vi "find_PrepLineObject_by_Name.vi"(9 "Name of Object":string, 10 "PrepLineObjects in":refnum<class "PrepLineObject.lvclass">[](array[class])) -> (0 "found PrepLineObject":refnum<class "PrepLineObject.lvclass">, 1 "instrument":string, 2 "selected array":bool[](array[boolean]), 3 "PrepLineObjectsOut":refnum<class "PrepLineObject.lvclass">[](array[class]), 4 "index of found":i32, 5 "found?":bool)   [LabVIEW 2017]
doc: "According to Name the correct PrepLineObject is located by looking through the Array of all PrepLineObjects (stored in a queue). The output array has the same size as the array with the switch objects and shows (state = true) the location of the Object that that has been selected. It also outputs the name of the instrument that belongs to the PrepLineObject that has changed"
uses:
  Classes/PrepLineObject/PrepLineObject.lvclass
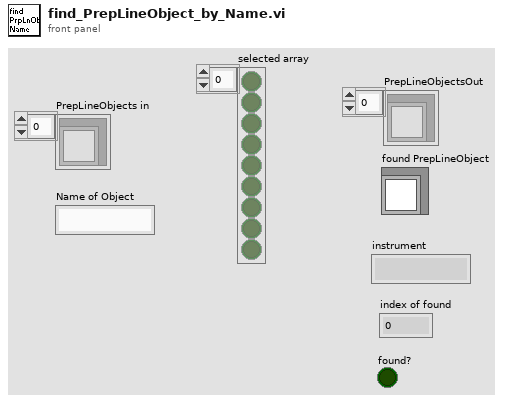
[diagram p1: front panel]
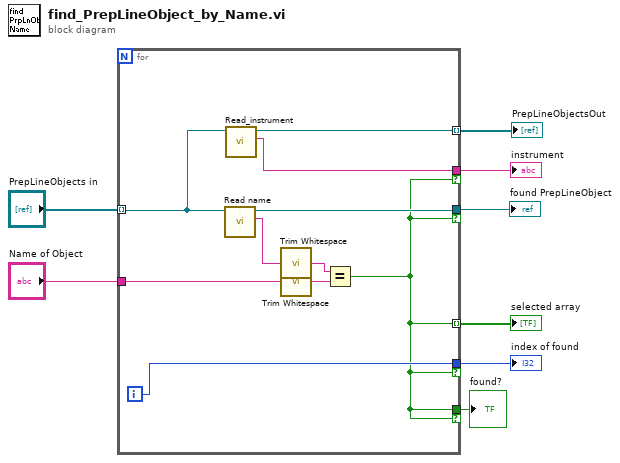
[diagram p0: block diagram]
diagram:
  n1 = for {
    tunnel: "PrepLineObjects in" -> [w13] mode=indexing
    tunnel: "Name of Object" -> [w17]
    tunnel: [w9] -> w7 mode=indexing
    tunnel: [w14] -> w6 if=w9
    tunnel: [w11] -> w5 if=w9
    tunnel: [w12] -> w3 mode=indexing
    tunnel: [w10] -> w2 if=w9
    tunnel: [w9] -> w1 if=w9
    i -> [w10]
    n2 = call-dynamic "Read name.vi"("PrepLineObject in"=w13) -> ("name"=w18:string, "PrepLineObject out"=w14:refnum<class "PrepLineObject.lvclass">)  [unwired: 8 in, 1 out]
    n3 = call-dynamic "Read_instrument.vi"("PrepLinePictureObjects in"=w13) -> ("PrepLinePictureObjects out"=w12:refnum<class "PrepLineObject.lvclass">, "instrument name"=w11:string)  [unwired: 7 in, 1 out]
    n4 = call <vilib>:"Trim Whitespace.vi"("string"=w18) -> ("trimmed string"=w15:string)  [unwired: 1 in]
    n5 = call <vilib>:"Trim Whitespace.vi"("string"=w17) -> ("trimmed string"=w16:string)  [unwired: 1 in]
    n6 = Equal?(x=w15, y=w16) -> (x = y?=w9:bool)
  }
  "selected array" <- w7
  "found PrepLineObject" <- w6
  "instrument" <- w5
  "PrepLineObjectsOut" <- w3
  "index of found" <- w2
  "found?" <- w1
